vi "Get Type Size.vi"(8 "error in (no error)":errorcluster, 11 "Channel Runtime in":refnum<class "Runtime.Channel.lvclass">) -> (0 "error out":errorcluster, 2 "size in bytes":u64, 3 "Channel Runtime out":refnum<class "Runtime.Channel.lvclass">)   [LabVIEW 2016, in "Data Sharing Framework.Runtime.lvlib" / "Runtime.Channel.lvclass"]
uses:
  Runtime.Channel.lvclass
  Runtime.Channel.lvclass/Runtime.Channel.ctl
  <vilib>/NI Veristand/VeriStand Data/VeriStand Data.lvlib
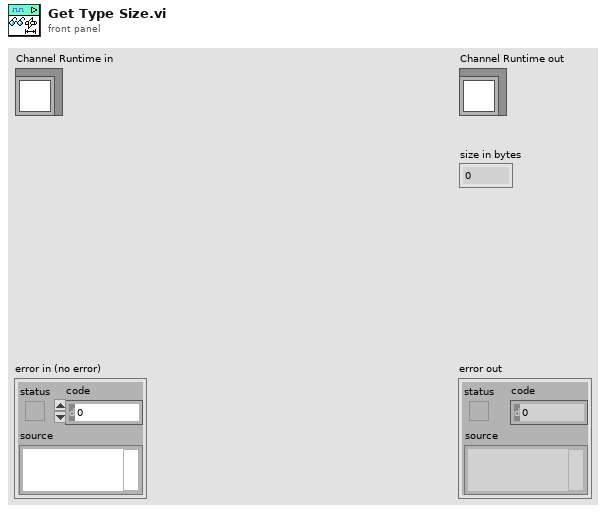
[diagram p1: front panel]
types:
  T1 = typedef "VeriStand Data.lvlib/Typedefs.Data Types.ctl" = enum16{"Boolean", "Single", "Double", "I8", "I16", "I32", "I64", "U8", "U16", "U32", "U64"}
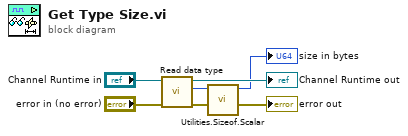
[diagram p0: block diagram]
diagram:
  n1 = call "Read data type.vi"("error in (no error)"="error in (no error)", "Runtime.Channel in"="Channel Runtime in") -> ("error out"=→"error out":errorcluster, "data type"=w5:T1, "Runtime.Channel out"=→"Channel Runtime out":refnum<class "Runtime.Channel.lvclass">)  [unwired: 7 in]
  n2 = call <vilib>:"Utilities.Sizeof.Scalar.vi"("data type"=w5) -> ("size in bytes"=→"size in bytes":u64)  [unwired: 9 in, 1 out]
